vi "GetPPMSItem_Example.vi"() -> ()   [LabVIEW 2019]
panel:
  in  "Channel":i32=1
  out "PPMS Data":sgl format="%#_8g"
  in  "Remote":bool
  in  "IP Address":string="127.0.0.1"
  # "Instrument Connection"
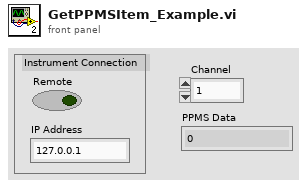
[diagram p1: front panel]
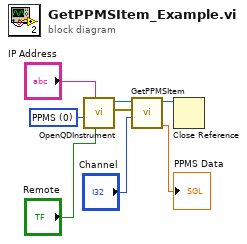
[diagram p0: block diagram]
diagram:
  w1 = 0 items=["PPMS", "VersaLab", "DynaCool", "SVSM"] ("Instrument Type")
  n1 = call "OpenQDInstrument.vi"("Remote"="Remote", "IP Address"="IP Address", "InstrumentType"=w1) -> ("error out"=w7:errorcluster, "Instrument Ref"=w8:refnum<k24>)  [unwired: 5 in]
  n2 = call "GetPPMSItem.vi"("Channel"="Channel", "error in (no error)"=w7, "Instrument Ref In"=w8) -> ("Result"=→"PPMS Data":dbl, "Instrument Ref Out"=w3:refnum<k24>)  [unwired: 1 in, 2 out]
  n3 = Close Reference(reference=w3) -> ()  [unwired: 1 in, 1 out]
